vi "FileGet.vi"(8 "error in (no error)":errorcluster, 10 "fileName":string, 11 "controller in":refnum<k24>) -> (0 "error out":errorcluster, 2 "GetFile":refnum<k24>, 3 "controller out":refnum<k24>)   [LabVIEW 2019]
uses:
  C:/Users/patrick/Documents/GitHub/Aerotech-Delay-Line/lvsrc/Aerotech-Ensemble-LabVIEW/2010-5.6/Bin/Aerotech.Ensemble.LabVIEW.dll
  Bin/Aerotech.Ensemble.LabVIEW.dll
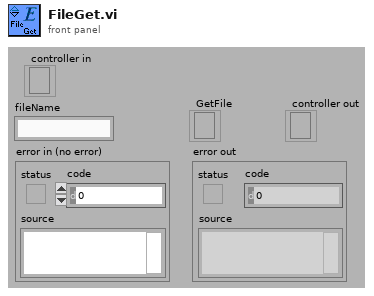
[diagram p1: front panel]
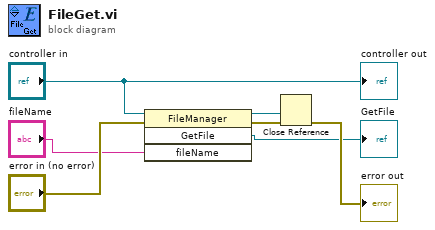
[diagram p0: block diagram]
diagram:
  n1 = invoke class="FileManager" method="GetFile"(reference="controller in", error in="error in (no error)", "fileName"="fileName") -> (reference out=w6:refnum<k24>, error out=w7:errorcluster, "GetFile"=→"GetFile":refnum<k24>)  [unwired: 1 in, 1 out]
  n2 = Close Reference(reference=w6, error in (no error)=w7) -> (error out=→"error out":errorcluster)
  "controller out" <- "controller in"
